vi "Create LokiHandler.vi"(4 "cookie file":path, 6 "Stream Fields Values":string[](array[string]), 7 "Stream Fields":string[](array[string]), 8 "error in":errorcluster, 9 "password":string, 10 "username":string, 11 "Loki Push URL":string="http://localhost:3100/loki/api/v1/push") -> (0 "error out":errorcluster, 3 "LokiHandler out":refnum<class "LokiHandler.lvclass">)   [LabVIEW 2017, in "hse-logger.lvlib" / "LokiHandler.lvclass"]
uses:
  LokiHandler.lvclass
  Formatter/LokiJsonFormatter/LokiJsonFormatter.lvclass
  LokiHandler.lvclass/LokiHandler.ctl
  <vilib>/httpClient/LabVIEWHTTPClient.lvlib
panel:
  # "Connector Pane"
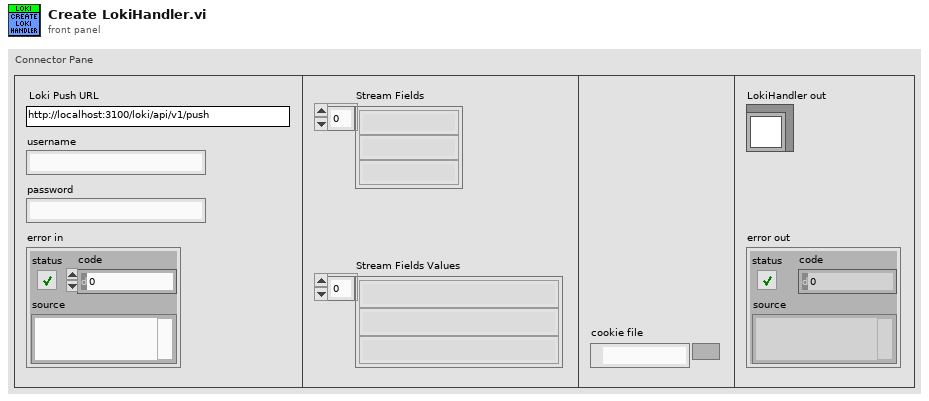
[diagram p1: front panel]
types:
  T1 = typedef "LabVIEWHTTPClient.lvlib/ClientHandle.ctl" = refnum<k1>
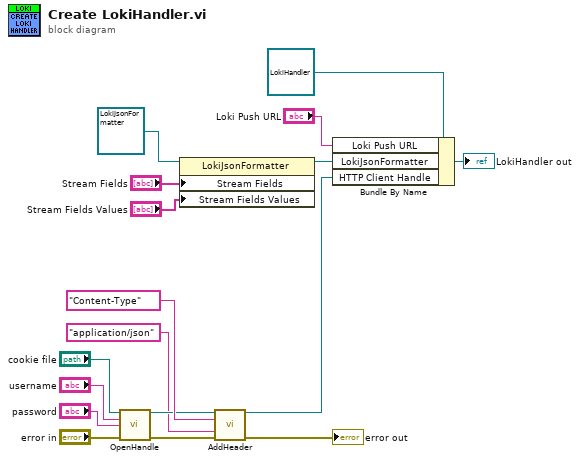
[diagram p0: block diagram]
diagram:
  n1 = call <vilib>:"OpenHandle.vi"("cookie file"="cookie file", "username"="username", "password"="password", "error in (no error)"="error in") -> ("client handle out"=w10:T1, "error out"=w11:errorcluster)  [unwired: 10 in]
  n2 = property class="LokiJsonFormatter"(reference=refnum<class "LokiJsonFormatter.lvclass"> refnum ("LokiJsonFormatter"), "Stream Fields"="Stream Fields", "Stream Fields Values"="Stream Fields Values") -> (reference out=w15:refnum<class "LokiJsonFormatter.lvclass">)  [unwired: 1 in, 1 out]
  n3 = call <vilib>:"AddHeader.vi"("client handle"=w10, "header"="Content-Type", "value"="application/json", "error in (no error)"=w11) -> ("client handle out"=w6:T1, "error out"=→"error out":errorcluster)  [unwired: 10 in]
  n4 = Bundle By Name(cluster=refnum<class "LokiHandler.lvclass"> refnum ("hse-logger.lvlib:LokiHandler.lvclass"), "Loki Push URL"="Loki Push URL", "LokiJsonFormatter"=w15, "HTTP Client Handle"=w6) -> (→"LokiHandler out":refnum<class "LokiHandler.lvclass">)
